vi "Read Display LE With binary conversion.vi"(0 "GEA2 Reference In":refnum<k24>, 5 "Standalone?":bool, 11 "Error In":errorcluster, 12 "Ignore Brightness":bool) -> (3 "Binary Number Displayed":u32, 4 "GEA2 Reference Out":refnum<k24>, 6 "Pass/Fail?":bool, 8 "Report Text":string, 10 "LEUI_LEDs_Out":T1, 15 "Error Out":errorcluster)   [LabVIEW 2016, in "2015 VA Washer.lvlib"]
doc: "This VI is used to verify the display on the LEUI."
uses:
  Projects/2015 VA Washer.lvlib
  C:/Automation/DLLs/PC Dot Net/GeaCommunication.dll
  controls/LEUI_LEDs.ctl
  Common/LabVIEW GEA2 Toolkit/LabVIEW_GEA2_Toolkit.lvlibp/type defs/Source_Destination.ctl
  Common/LabVIEW GEA2 Toolkit/LabVIEW_GEA2_Toolkit.lvlibp/type defs/ERD Read Data In.ctl
  Common/LabVIEW GEA2 Toolkit/LabVIEW_GEA2_Toolkit.lvlibp/type defs/Data Type.ctl
  Common/LabVIEW GEA2 Toolkit/LabVIEW_GEA2_Toolkit.lvlibp
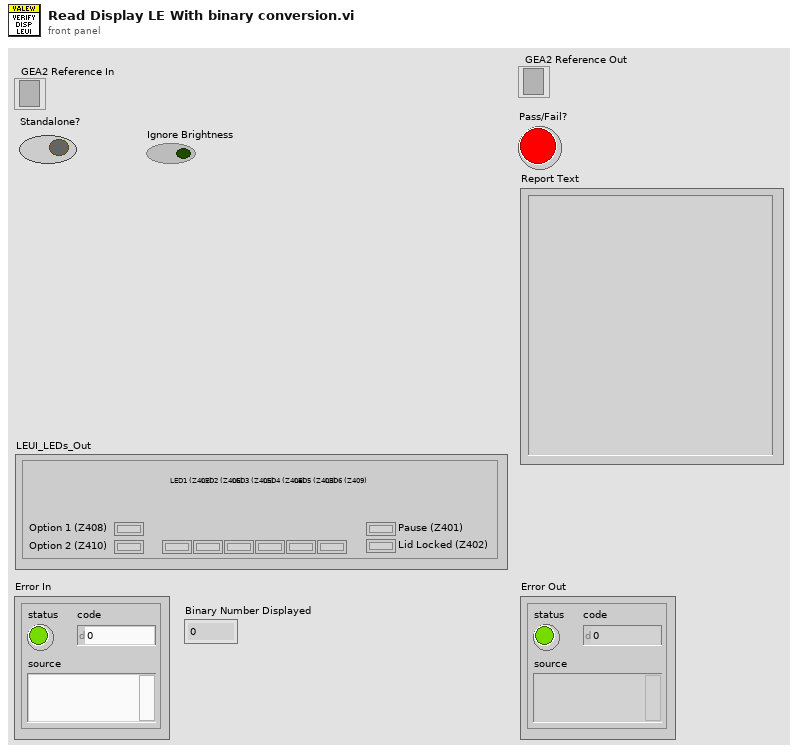
[diagram p1: front panel]
types:
  T1 = typedef "2015 VA Washer.lvlib/LEUI_LEDs.ctl" = cluster{"Pause (Z401)":bool, "Lid Locked (Z402)":bool, "LED1 (Z407)":bool, "LED2 (Z406)":bool, "LED3 (Z405)":bool, "LED4 (Z404)":bool, "LED5 (Z403)":bool, "LED6 (Z409)":bool, "Option 1 (Z408)":bool, "Option 2 (Z410)":bool}
  T2 = typedef "LabVIEW_GEA2_Toolkit.lvlibp/ERD Read Data In.ctl" = cluster{"ERD Number":u16, "Data Type":T3}
  T3 = typedef "LabVIEW_GEA2_Toolkit.lvlibp/Data Type.ctl" = enum16{"string", "boolean", "uint8_t", "uint16_t", "uint32_t", "uint64_t", "int8_t", "int16_t", "int32_t", "int64_t"}
  T4 = typedef "LabVIEW_GEA2_Toolkit.lvlibp/Source_Destination.ctl" = cluster{"Source":u8, "Destination":u8}
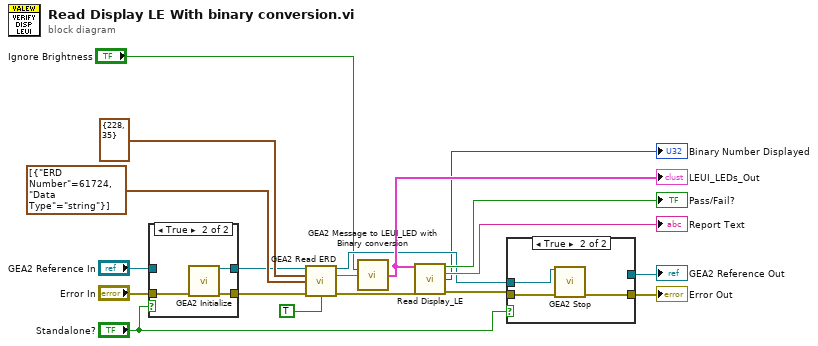
[diagram p0: block diagram]
diagram:
  n1 = case shown="True" "Standalone?" {
    tunnel: [w20 w24] -> w16
    tunnel: "Error In" -> [w20 w23]
    tunnel: [w21 w22] -> w14
    tunnel: "GEA2 Reference In" -> [w21 _]
    frame False {
    }
    frame True {
      n2 = call "GEA2 Initialize.vi"("error in"=w23) -> ("GEA2 Reference Out"=w22:refnum<k24>, "error out"=w24:errorcluster)  [unwired: 12 in, 1 out]
    }
  }
  n3 = call "GEA2 Read ERD.vi"("GEA2 Reference In"=w14, "GEA Inputs"=T4 {"Source"=228, "Destination"=35}, "Read ERD List"=T2[] [{"ERD Number"=61724, "Data Type"=enum."string"}], "Error In"=w16, "Verify ERD Response?"=TRUE) -> ("GEA2 Reference Out"=w3:refnum<k24>, "Raw Data Out"=w10:string, "Error Out"=w7:errorcluster)  [unwired: 7 in, 1 out]
  n4 = call "GEA2 Message to LEUI_LED with Binary conversion.vi"("Ignore Brightness"="Ignore Brightness", "Raw Data In"=w10) -> ("LEUI_LEDs"=w4:T1)  [unwired: 12 in, 1 out]
  "LEUI_LEDs_Out" <- w4
  n5 = call "Read Display_LE.vi"("LEUI_LEDs_Actual"=w4, "Error In"=w7) -> ("Pass/Fail?"=→"Pass/Fail?":bool, "Report Text"=→"Report Text":string, "Binary Number Displayed"=→"Binary Number Displayed":u32, "Error Out"=w6:errorcluster)  [unwired: 10 in]
  n6 = case shown="True" "Standalone?" {
    tunnel: w6 -> [w25 w29]
    tunnel: [w25 w28] -> w9
    tunnel: [w26 _] -> w5
    tunnel: w3 -> [w26 w27]
    frame False {
    }
    frame True {
      n7 = call "GEA2 Stop.vi"("GEA2 Reference In"=w27, "Error In"=w29) -> ("Error Out"=w28:errorcluster)  [unwired: 13 in]
    }
  }
  "GEA2 Reference Out" <- w5
  "Error Out" <- w9
